vi "TestStepsGui-Load.vi"(8 "error in":errorcluster, 10 "Data":T1={"BeginTS"=timestamp(0 s since 1904-01-01), "EndTS"=timestamp(0 s since 1904-01-01), "State"=enum."Init", "Status.Work"=enum."-", "Status.Process"=enum."-", "Status.Home"=enum."-", "Status.Wabco"=enum."-", "Status.Client"=enum."-", "BreakReason"=enum."-", "BreakSource"=enum."-", "DoorLock"=FALSE, "Status.Prod"=[], "UserAction"={"Stop"=FALSE, "Pause"=FALSE, "Next"=FALSE}, "UserData"={"GuiMode"=enum."Process", "Test"={"IgnoreResults"=FALSE, "IgnoreImages"=FALSE, "ServiceMode"=FALSE}, "ContinueOrder"=FALSE}, "Error"={"status"=FALSE, "code"=0, "source"=""}, "Code"={"Ready"=FALSE, "DoubleOrder"=FALSE, "OrderDone"=FALSE, "AllowSingleSlot"=FALSE, "CheckDM"=FALSE, "ThresholdA"=0, "ThresholdB"=0, "Plate"=enum."Wabco", "ImgPath"=path "", "Variant"={"State"=enum."Init", "ImgPath"=path "", "WabcoPlate"="", "WabcoProduct"="", "ClientProduct"="", "ClientPlate"="", "TotalQuantity"=0, "OrderQuantity"=0, "Serial"=0, "Wabco"={"LaserJob"="", "AdditionalTxt"="037", "FactoryCode"="", "RevID"=0, "ForkID"=0, "FailuresLimit"=0, "GlobalCnt"=0, "ScannerProgram"=0, "SerialFormat"=enum."6 dig", "CoordA"={"X"=0.0, "Y"=0.0, "Angle"=0.0}, "CoordB"={"X"=0.0, "Y"=0.0, "Angle"=0.0}, "DMCconfig"=0, "CVX_Program"=0}, "Client"={"LaserJob"="", "AdditionalTxt"="", "FactoryCode"="037", "RevID"=0, "ForkID"=0, "FailuresLimit"=0, "GlobalCnt"=0, "ScannerProgram"=0, "SerialFormat"=enum."6 dig", "CoordA"={"X"=0.0, "Y"=0.0, "Angle"=0.0}, "CoordB"={"X"=0.0, "Y"=0.0, "Angle"=0.0}, "DMCconfig"=0, "CVX_Program"=0}}}, "Rotations"=0, "ProdIdx"=0, "ProdDone"=[], "PrintedSerials-Wabco"=[], "PrintedSerials-Client"=[], "Counters-Wabco"={"Expected"=0, "Done"=0, "OK"=0, "NOK"=0, "NOKlimit"=0, "Part"=0, "PartOK"=0}, "Counters-Client"={"Expected"=0, "Done"=0, "OK"=0, "NOK"=0, "NOKlimit"=0, "Part"=0, "PartOK"=0}}) -> (0 "error out":errorcluster)   [LabVIEW 2016]
uses:
  Sequence/Sequence.Data.ctl
  Sequence/Sequence.State.ctl
  Sequence/Sequence.Step.Status.ctl
  Sequence/Sequence.Test.BreakReason.ctl
  Sequence/Sequence.Test.BreakSource.ctl
  Sequence/Sequence.Test.Status.ctl
  Sequence/Sequence.Slot.StatusData.ctl
  Sequence/Sequence.Test.Unload.Status.ctl
  Sequence/Sequence.Prod.StatusData.ctl
  Sequence/Sequence.UserActions.ctl
  Sequence/Sequence.UserData.ctl
  Sequence/Sequence.MainMode.ctl
  MainGui.TestOptions.ctl
  Sequence/Sequence.Code.Sets.ctl
  Sequence/Sequence.PlateType.ctl
  Logger/Logger.Variant.Sets.ctl
  Station/Station.Changeover.State.vi
  Station/Station.Plate.Properties.ctl
  Sequence/Sequence.Code.SerialFormat.ctl
  Drivers/V7310/LowLevel/V7310.Job.Sets.ctl
  Sequence/Sequence.Counters.ctl
  TestStepsGui.Action.ctl
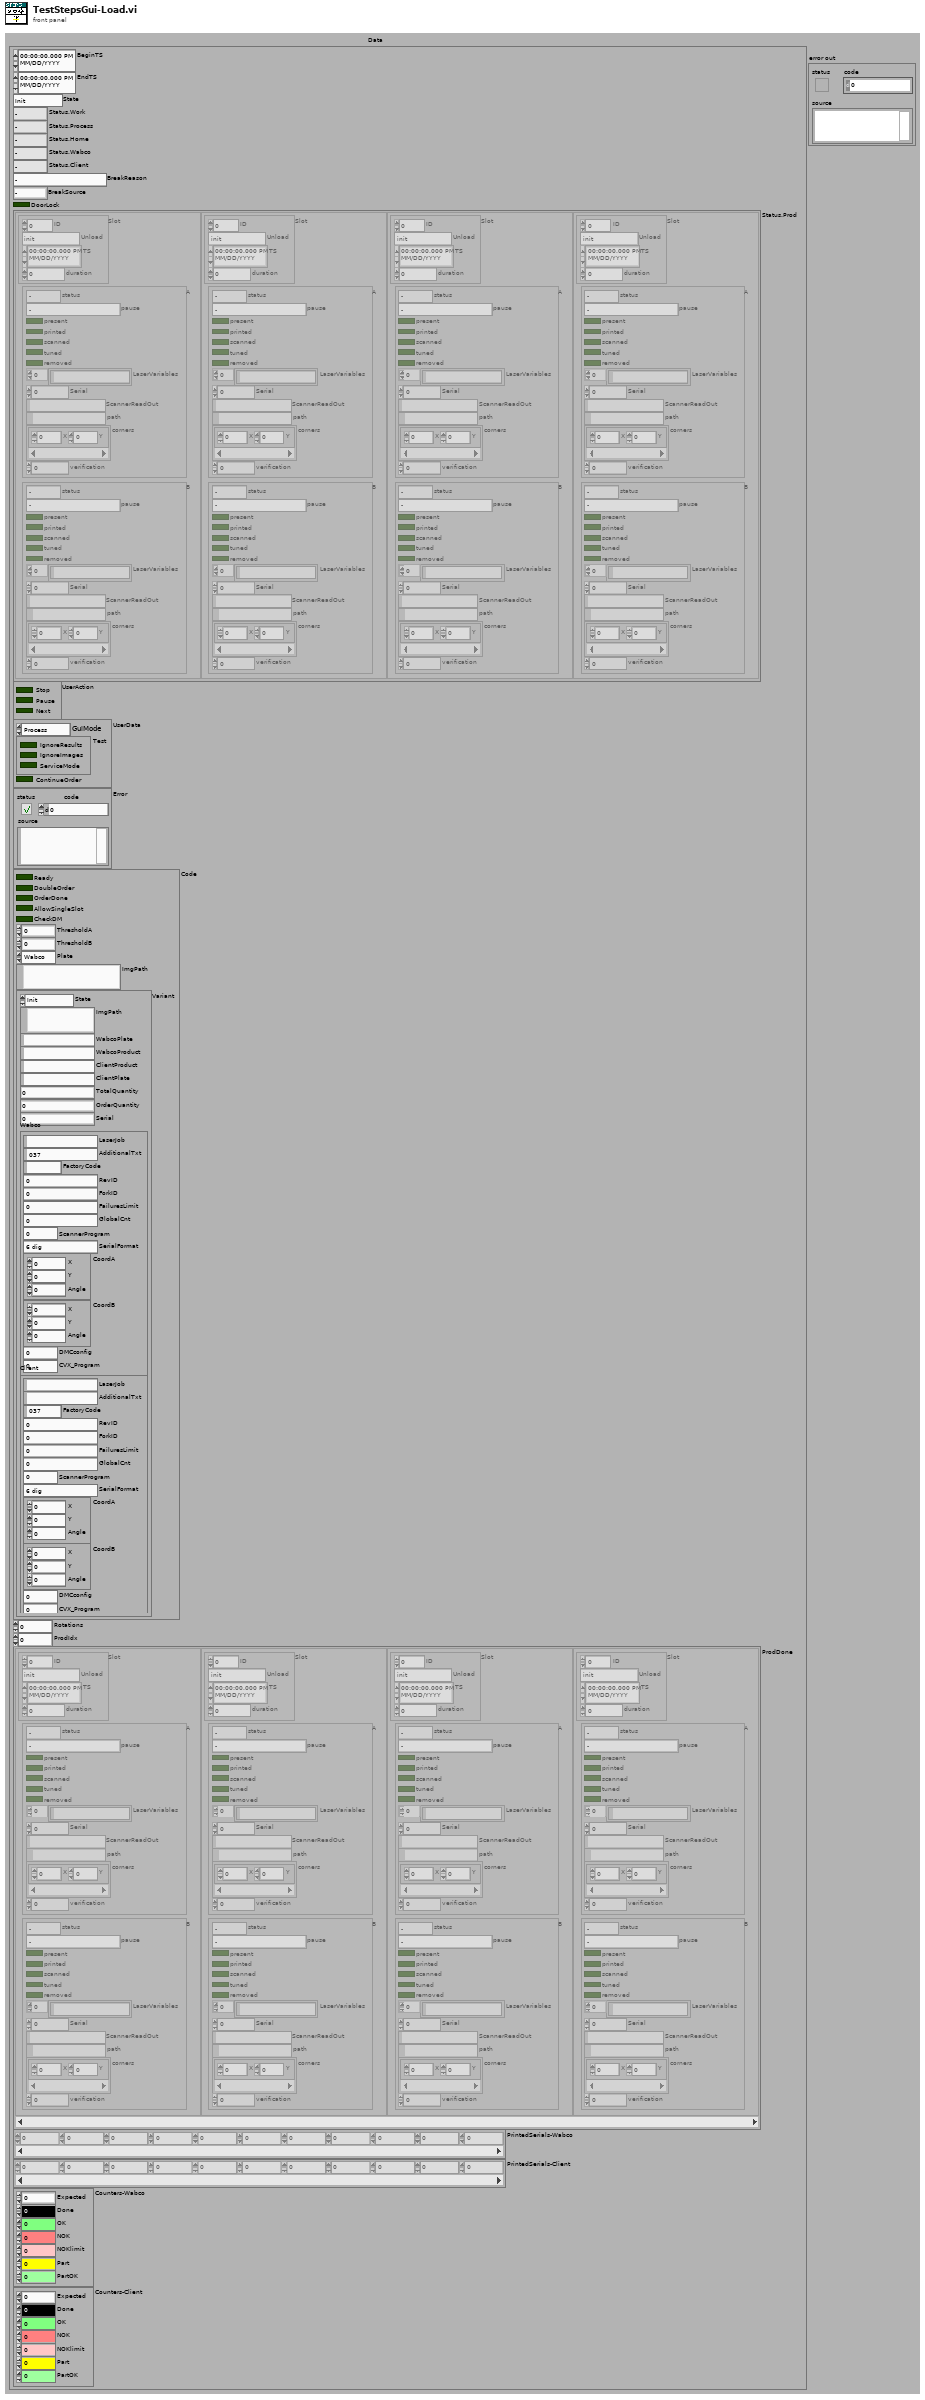
[diagram p1: front panel]
types:
  T1 = typedef "Sequence.Data.ctl" = cluster{"BeginTS":timestamp, "EndTS":timestamp, "State":T2, "Status.Work":T3, "Status.Process":T3, "Status.Home":T3, "Status.Wabco":T3, "Status.Client":T3, "BreakReason":T4, "BreakSource":T5, "DoorLock":bool, "Status.Prod":T6[], "UserAction":T10, "UserData":T11, "Error":errorcluster, "Code":T14, "Rotations":i32, "ProdIdx":i32, "ProdDone":T6[], "PrintedSerials-Wabco":i32[], "PrintedSerials-Client":i32[], "Counters-Wabco":T21, "Counters-Client":T21}
  T2 = typedef "Sequence.State.ctl" = enum16{"Init", "Idle", "Home", "Work", "Run", "Pause"}
  T3 = typedef "Sequence.Step.Status.ctl" = enum16{"-", "Pending", "Running", "Skipped", "Passed", "Failed", "Done", "Error", "Aborted", "Stopped"}
  T4 = typedef "Sequence.Test.BreakReason.ctl" = enum16{"-", "NOK container", "OK container", "Rev empty", "Rev missing", "Rev wrong", "Fork missing", "Fork wrong", "NOK limit", "Unload failure", "Single slot", "Part done", "Err: Prod move work", "Err: Prod move home", "Err: Prod lift work", "Err: Prod lift home", "Err: Prod Arm Work", "Err: Prod Arm NOK", "Err: Prod Arm OK", "Err: Prod NOK suck", "Err: Prod NOK drop", "Err: Prod OK missing", "Err: Prod OK suck", "Err: Prod OK drop"}
  T5 = typedef "Sequence.Test.BreakSource.ctl" = enum16{"-", "A", "B", "A/B"}
  T6 = typedef "Sequence.Test.Status.ctl" = cluster{"Slot":T7, "A":T9, "B":T9}
  T7 = typedef "Sequence.Slot.StatusData.ctl" = cluster{"ID":i32, "Unload":T8, "TS":timestamp, "duration":u32}
  T8 = typedef "Sequence.Test.Unload.Status.ctl" = enum16{"init", "check NOK", "check OK", "wait on NOK", "wait on OK", "wait on Unload", "done"}
  T9 = typedef "Sequence.Prod.StatusData.ctl" = cluster{"status":T3, "pause":T4, "present":bool, "printed":bool, "scanned":bool, "tuned":bool, "removed":bool, "LaserVariables":string[], "Serial":i32, "ScannerReadOut":string, "path":path, "corners":cluster{"X":i32, "Y":i32}[], "verification":u8}
  T10 = typedef "Sequence.UserActions.ctl" = cluster{"Stop":bool, "Pause":bool, "Next":bool}
  T11 = typedef "Sequence.UserData.ctl" = cluster{"GuiMode":T12, "Test":T13, "ContinueOrder":bool}
  T12 = typedef "Sequence.MainMode.ctl" = enum16{"Process", "Base", "Order", "Manual", "Logs", "Results", "Stats", "DMC Config"}
  T13 = typedef "MainGui.TestOptions.ctl" = cluster{"IgnoreResults":bool, "IgnoreImages":bool, "ServiceMode":bool}
  T14 = typedef "Sequence.Code.Sets.ctl" = cluster{"Ready":bool, "DoubleOrder":bool, "OrderDone":bool, "AllowSingleSlot":bool, "CheckDM":bool, "ThresholdA":u8, "ThresholdB":u8, "Plate":T15, "ImgPath":path, "Variant":T16}
  T15 = typedef "Sequence.PlateType.ctl" = enum16{"Wabco", "Client"}
  T16 = typedef "Logger.Variant.Sets.ctl" = cluster{"State":T17, "ImgPath":path, "WabcoPlate":string, "WabcoProduct":string, "ClientProduct":string, "ClientPlate":string, "TotalQuantity":u16, "OrderQuantity":u16, "Serial":i32, "Wabco":T18, "Client":T18}
  T17 = typedef "Station.Changeover.State.vi" = enum16{"Init", "Scaning", "NOK", "Wait for ack", "Ready"}
  T18 = typedef "Station.Plate.Properties.ctl" = cluster{"LaserJob":string, "AdditionalTxt":string, "FactoryCode":string, "RevID":u8, "ForkID":u8, "FailuresLimit":u16, "GlobalCnt":i32, "ScannerProgram":u8, "SerialFormat":T19, "CoordA":T20, "CoordB":T20, "DMCconfig":i32, "CVX_Program":u16}
  T19 = typedef "Sequence.Code.SerialFormat.ctl" = enum8{"", "6 dig", "7 dig"}
  T20 = typedef "V7310.Job.Sets.ctl" = cluster{"X":dbl, "Y":dbl, "Angle":dbl}
  T21 = typedef "Sequence.Counters.ctl" = cluster{"Expected":u16, "Done":u16, "OK":u16, "NOK":u16, "NOKlimit":u16, "Part":u16, "PartOK":u16}
  T22 = typedef "TestStepsGui.Action.ctl" = enum32{"idle", "constructor", "destructor", "--- TestStepsGui ---", "Select", "Load", "Start", "Update", "Update Images"}
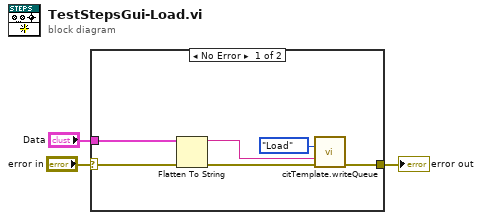
[diagram p0: block diagram]
diagram:
  n1 = case shown="No Error" "error in" {
    selector: "error in" -> [w8 w10]
    tunnel: [w9 w10] -> w2
    tunnel: "Data" -> [w4 _]
    frame No Error {
      n2 = Flatten To String(anything=w4, error in (no error)=w8) -> (data string=w5:string, error out=w6:errorcluster)  [unwired: 2 in, 1 out]
      n3 = call "citTemplate.writeQueue.vi"("event in (if not connected:all statemachine with data event)"=TestStepsGui.Action."Load" ("Action"), "data in"=w5, "error in (no error)"=w6) -> ("error out"=w9:errorcluster)  [unwired: 12 in]
    }
    frame Error {
    }
  }
  "error out" <- w2
